vi "App Init.vi"(8 "error in (no error)":errorcluster, 10 "Core APIs":T1, 11 "DemoApp in":refnum<class "DemoApp.lvclass">) -> (0 "error out":errorcluster, 3 "DemoApp out":refnum<class "DemoApp.lvclass">)   [LabVIEW 2020, in "VolatusDemo.lvlib" / "DemoApp.lvclass"]
uses:
  DemoApp.lvclass
  Volatus/Core APIs.ctl
  Volatus/VolatusAPI/VolatusAPI.lvclass
  Volatus/Event API/EventAPI.lvclass
  DemoApp.lvclass/DemoApp.ctl
  Volatus/Volatus.lvlib
  Volatus/TelemetryAPI/TelemetryAPI.lvclass
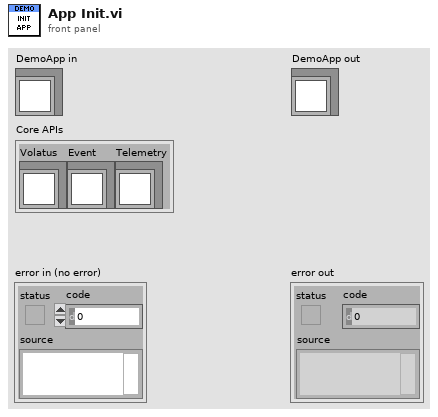
[diagram p1: front panel]
types:
  T1 = typedef "Volatus.lvlib/Core APIs.ctl" = cluster{"Volatus":refnum<class "VolatusAPI.lvclass">, "Event":refnum<class "EventAPI.lvclass">, "Telemetry":refnum<class "TelemetryAPI.lvclass">}
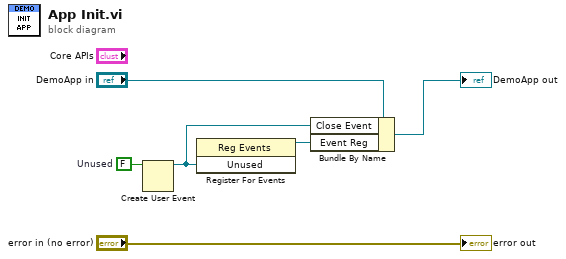
[diagram p0: block diagram]
diagram:
  w4 = FALSE  # Unused
  n1 = Create User Event(user event datatype=w4) -> (user event=w1:refnum<user-event>)  [unwired: 1 in, 1 out]
  n2 = register-events(w1) -> (reference out=w2:refnum<event-registration>)  [unwired: 2 in, 1 out]
  n3 = Bundle By Name(cluster="DemoApp in", "Close Event"=w1, "Event Reg"=w2) -> (→"DemoApp out":refnum<class "DemoApp.lvclass">)
  "error out" <- "error in (no error)"
